vi "Read Header and Footer [ ].vi"(8 "error in (no error)":errorcluster, 11 "Header and Footer Class in":refnum<class "Header and Footer Class.lvclass">) -> (0 "error out":errorcluster, 2 "Header and Footer [ ]":T1[](array[typedef]), 3 "Header and Footer Class out":refnum<class "Header and Footer Class.lvclass">)   [LabVIEW 2019, in "Exaprom PDF.lvlib" / "Header and Footer Class.lvclass"]
uses:
  Header and Footer Class.lvclass
  Controls/Header Footer cluster V2.ctl
  Controls/Header, Footer and Watermark Controls/Header or Footer.ctl
  Controls/Header, Footer and Watermark Controls/Header Footer Type.ctl
  Controls/Header, Footer and Watermark Controls/Header footer horiz alignment.ctl
  Controls/Table Controls/Cell Vertical alignment.ctl
  Controls/Text Controls/Line spacing.ctl
  Controls/Header, Footer and Watermark Controls/Page number.ctl
  Controls/Font Controls/Font complete cluster horizontal.ctl
  Controls/Font Controls/Font size.ctl
  Controls/Font Controls/Font color.ctl
  Controls/Font Controls/Type and encoding.ctl
  Controls/Text Controls/Unicode/Type and run direction.ctl
  C:/work/niobrara_lv/labview pdf writer fixing/DLL/itextsharp.dll
  DLL/itextsharp.dll
  Controls/Header, Footer and Watermark Controls/Header Footer Line.ctl
  Header and Footer Class.lvclass/Header and Footer Class.ctl
  Exaprom PDF.lvlib
panel:
  # "X"
  # "Y"
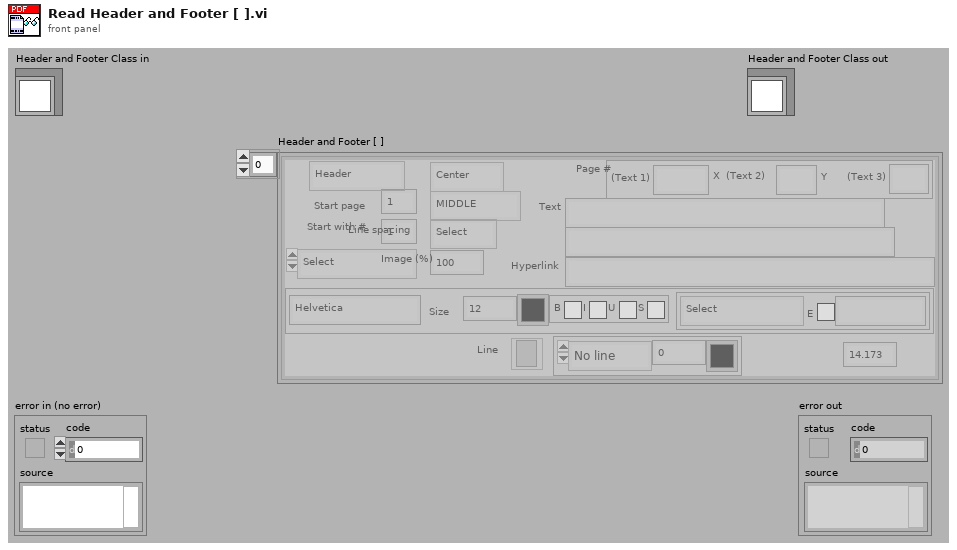
[diagram p1: front panel]
types:
  T1 = typedef "Header Footer cluster V2.ctl" = cluster{"Header or Footer":T2, "Start page":i32, "Start with #":i32, "Type":T3, "Alignment":T4, "Vertical Alignement":T5, "Line spacing":T6, "Image (%)":sgl, "Page #":T7, "Text":string, "Path":string, "Font":T8, "Font refnum":refnum<k24>, "Line":cluster{"Line":T13, "Thickness (points)":sgl, "Colour":T10}, "Vert margin":dbl, "Hyperlink":string}
  T2 = typedef "Exaprom PDF.lvlib/Header or Footer.ctl" = enum16{"Header", "Footer"}
  T3 = typedef "Exaprom PDF.lvlib/Header Footer Type.ctl" = enum16{"Select", "Text", "Text + hyperlink", "Page number", "Image", "Image + hyperlink"}
  T4 = typedef "Exaprom PDF.lvlib/Header footer horiz alignment.ctl" = enum16{"Left", "Center", "Right"}
  T5 = typedef "Exaprom PDF.lvlib/Cell Vertical alignment.ctl" = enum16{"TOP", "MIDDLE", "BOTTOM"}
  T6 = typedef "Exaprom PDF.lvlib/Line spacing.ctl" = enum16{"Select", "1.0", "1.5", "2.0"}
  T7 = typedef "Exaprom PDF.lvlib/Page number.ctl" = cluster{"Text 1":string, "Text 2":string, "Text 3":string}
  T8 = typedef "Exaprom PDF.lvlib/Font complete cluster horizontal.ctl" = cluster{"Name":string, "Size":T9, "Color":T10, "Style":cluster{"Bold":bool, "Italic":bool, "Underline":bool, "Strikeout":bool}, "Type":T11}
  T9 = typedef "Exaprom PDF.lvlib/Font size.ctl" = sgl
  T10 = typedef "Exaprom PDF.lvlib/Font color.ctl" = u32
  T11 = typedef "Exaprom PDF.lvlib/Type and encoding.ctl" = cluster{"Type&direction":T12, "Embedded":bool, "Encoding":string}
  T12 = typedef "Exaprom PDF.lvlib/Type and run direction.ctl" = enum16{"Select", "ASCII", "UTF-16", "UTF-16 (default)", "UTF-16 (LTR)", "UTF-16 (RTL)"}
  T13 = typedef "Exaprom PDF.lvlib/Header Footer Line.ctl" = enum16{"No line", "Horizontal line"}
  T14 = typedef "Header Footer [ ] V2.ctl" = T1[]
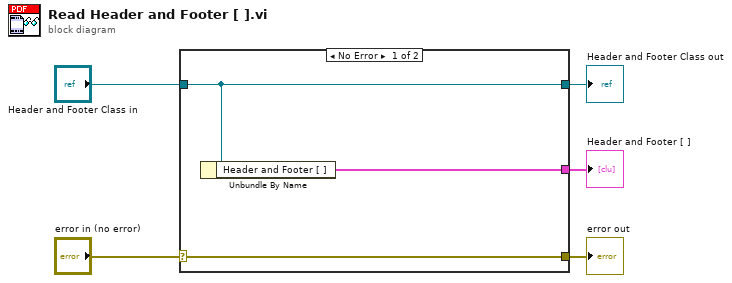
[diagram p0: block diagram]
diagram:
  n1 = case shown="No Error" "error in (no error)" {
    selector: "error in (no error)" -> [w8 w9]
    tunnel: [w8 w9] -> w4
    tunnel: [w7 w10] -> w2
    tunnel: "Header and Footer Class in" -> [w7 w10]
    tunnel: [w6 _] -> w1
    frame No Error {
      n2 = Unbundle By Name(w7) -> ("Header and Footer [ ]"=w6:T14)
    }
    frame Error {
    }
  }
  "error out" <- w4
  "Header and Footer Class out" <- w2
  "Header and Footer [ ]" <- w1
